vi "SLL DAQ ENGINE VI Tree.vi"   [LabVIEW 2009]
uses:
  Sub VIs/DAQ Engine/Controls/SLL DE List of AI Channel Type.ctl
  Sub VIs/DAQ Engine/Controls/SLL DE List of Analog Inputs.ctl
  Sub VIs/DAQ Engine/Controls/SLL DE List of Analog Outputs.ctl
  Sub VIs/DAQ Engine/Controls/SLL DE List of Digital Inputs.ctl
  Sub VIs/DAQ Engine/Controls/SLL DE List of Digital Outputs.ctl
panel:
  # "SEE DIAGRAM FOR VI HIERARCHY\n\nTHE DIAGRAM OF THIS VI CONTAINS ALL THE USER-LEVEL VIS\nFOR THE NI-SWITCH INSTRUMENT DRIVER.  USER-LEVEL VIS ARE TYPICALLY THE ONLY \nVIS THAT USERS NEED TO CALL TO CONTROL DAQ.  THE HIERARCHY ILLUSTRATES\nTHE STRUCTURE OF THE DAQ ENGINE AND THE ORGANIZATION OF VIS."
types:
  T1 = typedef "SLL DE List of AI Channel Type.ctl" = enum16{"Pressure", "Flow", "Temperature", "Time Scale", "Voltage", "Current", "Frequency", "Sound", "Speed", "Torque", "Distance", "Channel Type 1", "Channel Type 2", "Channel Type 3"}
  T2 = typedef "SLL DE List of Analog Inputs.ctl" = enum16{"None"}
  T3 = typedef "SLL DE List of Analog Outputs.ctl" = enum16{"None"}
  T4 = typedef "SLL DE List of Digital Inputs.ctl" = enum16{"STATION1_START", "STATION1_STOP", "STATION1_CLAMPED", "STATION1_TC_PASS", "STATION1_TC_FAIL", "STATION2_START", "STATION2_STOP", "STATION2_CLAMPED", "STATION2_TC_PASS", "STATION2_TC_FAIL", "STATION3_START", "STATION3_STOP", "STATION3_CLAMPED", "STATION3_TC_PASS", "STATION3_TC_FAIL", "STATION4_START", "STATION4_STOP", "STATION4_CLAMPED", "STATION4_TC_PASS", "STATION4_TC_FAIL"}
  T5 = typedef "SLL DE List of Digital Outputs.ctl" = enum16{"STATION1_START TEST", "STATION1_STOP TEST", "STATION1_LIGHT1", "STATION1_LIGHT2", "STATION1_LIGHT3", "STATION2_START TEST", "STATION2_STOP TEST", "STATION2_LIGHT1", "STATION2_LIGHT2", "STATION2_LIGHT3", "STATION3_START TEST", "STATION3_STOP TEST", "STATION3_LIGHT1", "STATION3_LIGHT2", "STATION3_LIGHT3", "STATION4_START TEST", "STATION4_STOP TEST", "STATION4_LIGHT1", "STATION4_LIGHT2", "STATION4_LIGHT3"}
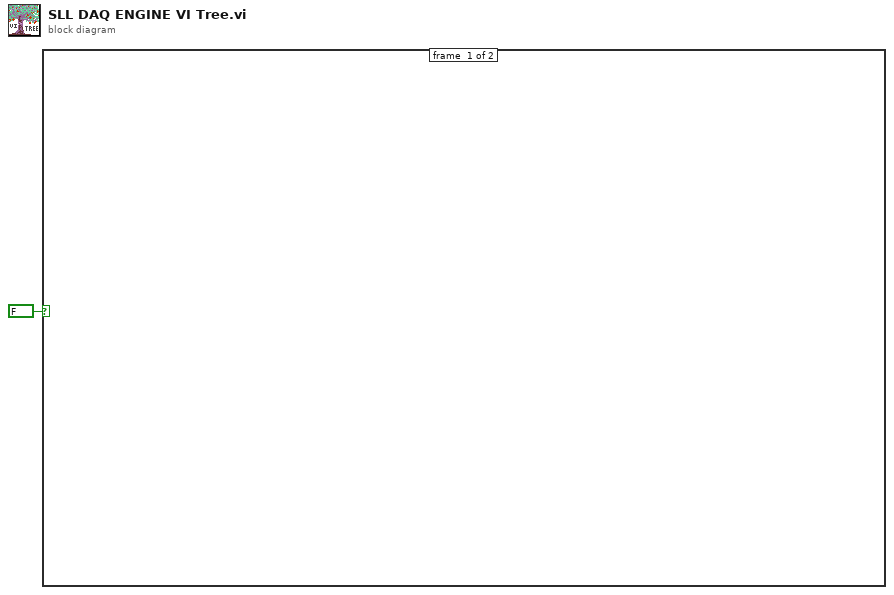
[diagram p0: block diagram]
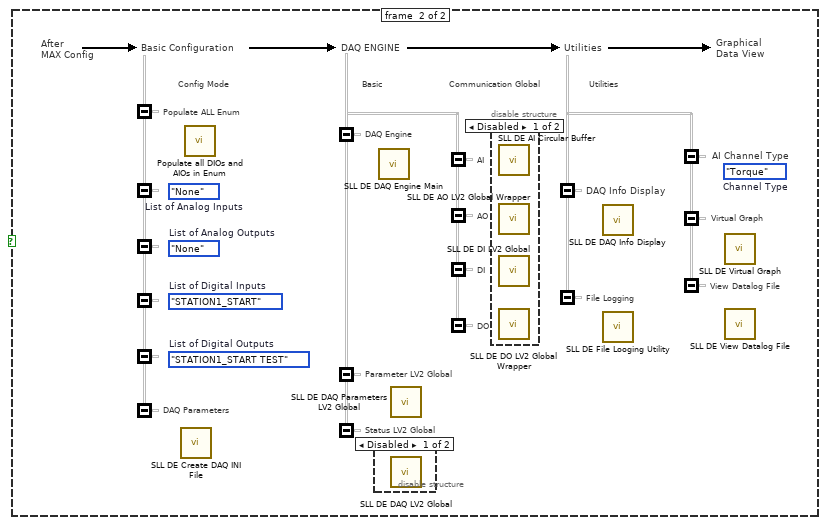
[diagram p2: hidden frame]
diagram:
  n1 = case shown="True" FALSE {
    frame #0 {
    }
    frame #1 {
      (unwired) SLL_DE_List_of_AI_Channel_Type."Torque"  # Channel Type
      (unwired) SLL_DE_List_of_Analog_Inputs."None"  # List of Analog Inputs
      (unwired) SLL_DE_List_of_Analog_Outputs."None"  # List of Analog Outputs
      (unwired) SLL_DE_List_of_Digital_Inputs."STATION1_START"  # List of Digital Inputs
      (unwired) SLL_DE_List_of_Digital_Outputs."STATION1_START TEST"  # List of Digital Outputs
      # "DAQ ENGINE"
      # "View Datalog File"
      # "AI Channel Type"
      # "Virtual Graph"
      # "Utilities"
      # "DO"
      # "DI"
      # "AO"
      # "AI"
      # "DAQ Parameters"
      # "Status LV2 Global"
      # "Parameter LV2 Global"
      # "DAQ Engine"
      # "Basic"
      # "Populate ALL Enum"
      # "Communication Global"
      # "Config Mode"
      # "Utilities"
      # "Basic Configuration"
      # "File Logging"
      # "DAQ Info Display"
      # "Graphical\nData View"
      # "After \nMAX Config"
      n2 = call "SLL DE Create DAQ INI File.vi"() -> ()  [unwired: 11 in, 1 out]
      n3 = call "Populate all DIOs and AIOs in Enum.vi"() -> ()  [unwired: 11 in, 1 out]
      n4 = disable-structure shown="Disabled" {
        frame #0 {
          n5 = call "SLL DE DAQ LV2 Global.vi"() -> ()  [unwired: 9 in, 3 out]
        }
        frame #1 {
        }
      }
      n6 = call "SLL DE DAQ Engine Main.vi"() -> ()  [unwired: 11 in, 1 out]
      n7 = call "SLL DE DAQ Parameters LV2 Global.vi"() -> ()  [unwired: 10 in, 2 out]
      n8 = disable-structure shown="Disabled" {
        frame #0 {
          n9 = call "SLL DE AI Circular Buffer.vi"() -> ()  [unwired: 6 in, 6 out]
          n10 = call "SLL DE AO LV2 Global Wrapper.vi"() -> ()  [unwired: 8 in, 4 out]
          n11 = call "SLL DE DI LV2 Global.vi"() -> ()  [unwired: 8 in, 4 out]
          n12 = call "SLL DE DO LV2 Global Wrapper.vi"() -> ()  [unwired: 8 in, 4 out]
        }
        frame #1 {
        }
      }
      n13 = call "SLL DE DAQ Info Display.vi"() -> ()  [unwired: 11 in, 1 out]
      n14 = call "SLL DE File Looging Utility.vi"() -> ()  [unwired: 11 in, 1 out]
      n15 = call "SLL DE Virtual Graph.vi"() -> ()  [unwired: 11 in, 1 out]
      n16 = call "SLL DE View Datalog File.vi"() -> ()  [unwired: 11 in, 1 out]
    }
  }
